vi "ReadOrDestroyStream.vi"(7 "EndpointName":string, 8 "error in (no error)":errorcluster, 9 "Connected":bool, 10 "IP Address":string, 11 "endpoint in":refnum<k21>) -> (0 "error out":errorcluster, 2 "Array":T1[](array[typedef]), 3 "endpoint Out":refnum<k21>)   [LabVIEW 2018]
uses:
  Controls/Clusts/StreamReceiveClust.ctl
  Controls/Enums/StreamReceiveStates.ctl
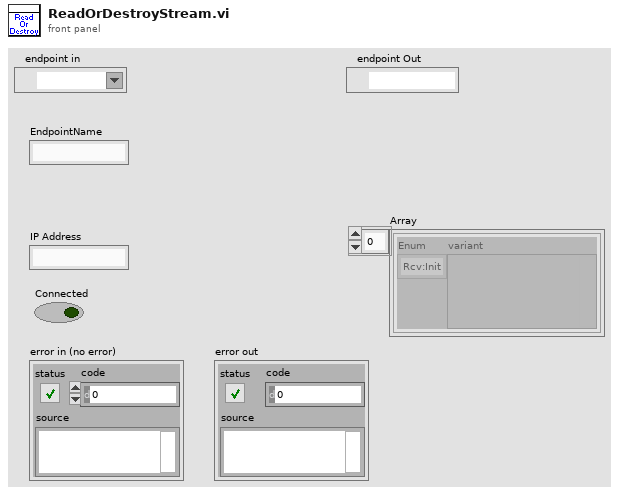
[diagram p1: front panel]
types:
  T1 = typedef "StreamReceiveClust.ctl" = cluster{"Enum":T2, "variant":variant}
  T2 = typedef "StreamReceiveStates.ctl" = enum16{"Rcv:Init", "Rcv:Read", "Rcv:Log", "Rcv:FromMast", "Rcv:FromSlav"}
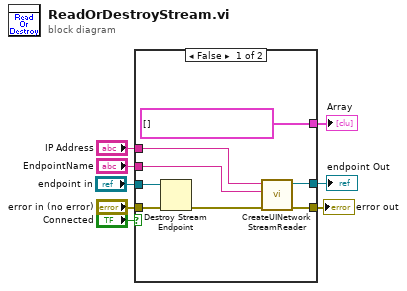
[diagram p0: block diagram]
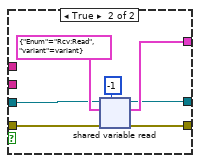
[diagram p2: hidden frame]
diagram:
  n1 = case shown="False" "Connected" {
    tunnel: [w16 w22] -> w5
    tunnel: "error in (no error)" -> [w15 w23]
    tunnel: "IP Address" -> [w13 _]
    tunnel: "EndpointName" -> [w11 _]
    tunnel: [cluster{"Enum":T2, "variant":variant}[] [] w19] -> w3
    tunnel: [w10 w18] -> w1
    tunnel: "endpoint in" -> [w9 w17]
    frame False {
      n2 = Destroy Stream Endpoint(8:w15, 11:w9) -> (0:w14:errorcluster)
      n3 = call "CreateUINetworkStreamReader.vi"("ErrorIn"=w14, "ReaderName"=w11, "IPAddress"=w13) -> ("ErrorOut"=w16:errorcluster, "reader endpoint"=w10:refnum<k21>)  [unwired: 7 in]
    }
    frame True {
      n4 = shared-variable-read(w17, w23, -1 ("# elements"), T1 {"Enum"=enum."Rcv:Read", "variant"=variant}) -> (w18:refnum<k21>, w22:errorcluster, w19:T1[])  [unwired: 1 in, 1 out]
    }
  }
  "error out" <- w5
  "Array" <- w3
  "endpoint Out" <- w1
